vi "Write To String Delimiter.vi"(8 "error in (no error)":errorcluster, 10 "Delimiter":string, 11 "Abs_Double Float 1D in":refnum<class "Abs_Complex Double Float 1D.lvclass">) -> (0 "error out":errorcluster, 3 "Abs_Double Float 1D out":refnum<class "Abs_Complex Double Float 1D.lvclass">)   [LabVIEW 2019, in "Abs_Complex Double Float 1D.lvclass"]
uses:
  Abs_Complex Double Float 1D.lvclass
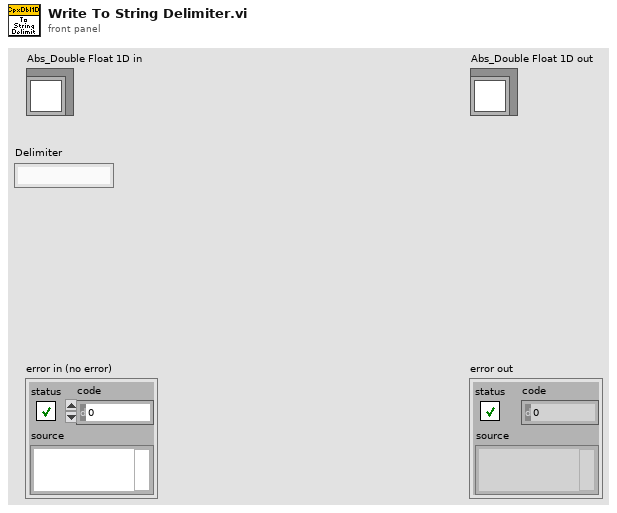
[diagram p1: front panel]
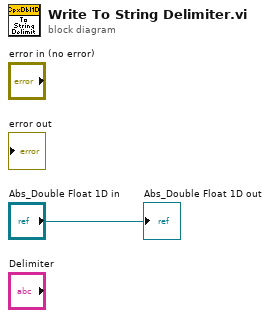
[diagram p0: block diagram]
diagram:
  "Abs_Double Float 1D out" <- "Abs_Double Float 1D in"
